vi "macro_TrajectoryConstraint_MaxVel.vi"   [LabVIEW 2019, in "Trajectory_Library.lvlib"]
uses:
  Trajectory_Library.lvlib
  Enum/TRAJECTORY_SPLINE_TYPE_ENUM.ctl
types:
  T1 = typedef "Trajectory_Library.lvlib/TRAJECTORY_SPLINE_TYPE_ENUM.ctl" = enum16{"Cubic", "Cubic With Weights", "Quintic", "Quintic With Weights"}
  T2 = typedef "Trajectory_Library.lvlib/WEIGHTED_WAYPOINT.ctl" = cluster{"TRANSLATION":T3, "ROTATION":T4, "SCALAR":dbl}
  T3 = typedef "Trajectory_Library.lvlib/TRANSLATION2D.ctl" = cluster{"X":dbl, "Y":dbl}
  T4 = typedef "Trajectory_Library.lvlib/ROTATION2D.ctl" = cluster{"VALUE":dbl, "COS":dbl, "SIN":dbl}
  T5 = typedef "Trajectory_Library.lvlib/TRAJ_CONFIG.ctl" = cluster{"MaxVelocity":dbl, "Max Acceleration":dbl, "StartVelocity":dbl, "End Velocity":dbl, "Reversed":bool, "Constraints":variant[]}
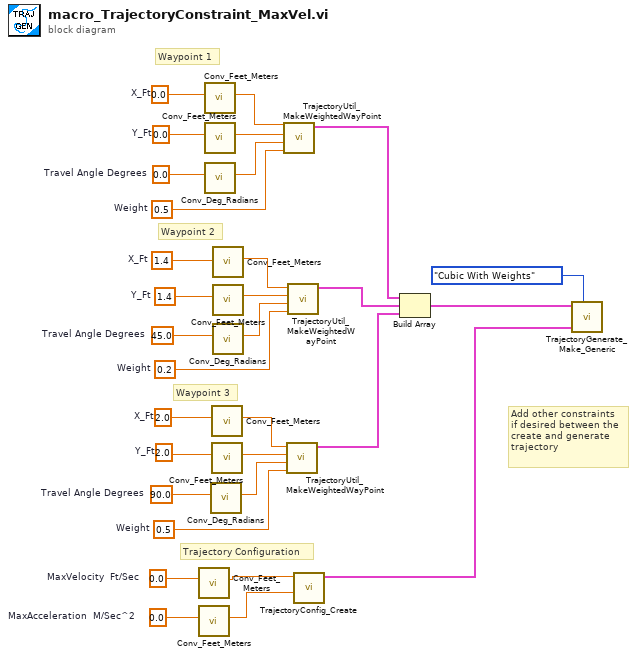
[diagram p0: block diagram]
diagram:
  w6 = 2.0  # X_Ft
  w5 = 2.0  # Y_Ft
  w18 = 90.0  # Travel Angle Degrees
  w25 = 0.5  # Weight
  w10 = 1.4  # X_Ft
  w9 = 1.4  # Y_Ft
  w20 = 45.0  # Travel Angle Degrees
  w26 = 0.2  # Weight
  w14 = 0.0  # X_Ft
  w13 = 0.0  # Y_Ft
  w21 = 0.0  # Travel Angle Degrees
  w27 = 0.5  # Weight
  w2 = 0.0  # MaxVelocity  Ft/Sec
  w1 = 0.0  # MaxAcceleration  M/Sec^2
  # "Trajectory Configuration"
  # "Waypoint 3"
  # "Waypoint 2"
  # "Waypoint 1"
  # "Add other constraints\nif desired between the\ncreate and generate\ntrajectory"
  n1 = call "Conv_Feet_Meters.vi"("Feet"=w2) -> ("Meters"=w4:dbl)  [unwired: 10 in]
  n2 = call "Conv_Feet_Meters.vi"("Feet"=w1) -> ("Meters"=w3:dbl)  [unwired: 10 in]
  n3 = call "Conv_Feet_Meters.vi"("Feet"=w14) -> ("Meters"=w15:dbl)  [unwired: 10 in]
  n4 = call "Conv_Feet_Meters.vi"("Feet"=w13) -> ("Meters"=w16:dbl)  [unwired: 10 in]
  n5 = call "Conv_Deg_Radians.vi"("Degress"=w21) -> ("Radians"=w22:dbl)  [unwired: 10 in]
  n6 = call "Conv_Deg_Radians.vi"("Degress"=w18) -> ("Radians"=w17:dbl)  [unwired: 10 in]
  n7 = call "Conv_Feet_Meters.vi"("Feet"=w6) -> ("Meters"=w7:dbl)  [unwired: 10 in]
  n8 = call "Conv_Feet_Meters.vi"("Feet"=w5) -> ("Meters"=w8:dbl)  [unwired: 10 in]
  n9 = call "Conv_Feet_Meters.vi"("Feet"=w10) -> ("Meters"=w11:dbl)  [unwired: 10 in]
  n10 = call "Conv_Feet_Meters.vi"("Feet"=w9) -> ("Meters"=w12:dbl)  [unwired: 10 in]
  n11 = call "Conv_Deg_Radians.vi"("Degress"=w20) -> ("Radians"=w19:dbl)  [unwired: 10 in]
  n12 = call "TrajectoryUtil_MakeWeightedWayPoint.vi"("Weight"=w27, "Travel Angle Radians"=w22, "Y_M"=w16, "X_M"=w15) -> ("WEIGHTED_WAYPOINT"=w31:T2)  [unwired: 7 in]
  n13 = call "TrajectoryUtil_MakeWeightedWayPoint.vi"("Weight"=w25, "Travel Angle Radians"=w17, "Y_M"=w8, "X_M"=w7) -> ("WEIGHTED_WAYPOINT"=w23:T2)  [unwired: 7 in]
  n14 = call "TrajectoryUtil_MakeWeightedWayPoint.vi"("Weight"=w26, "Travel Angle Radians"=w19, "Y_M"=w12, "X_M"=w11) -> ("WEIGHTED_WAYPOINT"=w24:T2)  [unwired: 7 in]
  n15 = call "TrajectoryConfig_Create.vi"("MaxAcceleration"=w3, "MaxVelocity"=w4) -> ("TRAJECTORY_CONFIG"=w28:T5)  [unwired: 9 in]
  n16 = Build Array(w31, w24, w23) -> (w30:T2[])
  n17 = call "TrajectoryGenerate_Make_Generic.vi"("Spline Type"=TRAJECTORY_SPLINE_TYPE_ENUM."Cubic With Weights", "traj_config"=w28, "WeightedWayPoints"=w30) -> ()  [unwired: 7 in, 2 out]
